vi "Read_Instr.vi"(8 "error in (no error)":errorcluster caption="entrée d'erreur (pas d'erreur)", 11 "Class Instrument Multimeter en entrée":refnum<class "Class Instrument Spectrum_Analyser.lvclass">) -> (0 "error out":errorcluster caption="sortie d'erreur", 3 "Class Instrument Multimeter en sortie":refnum<class "Class Instrument Spectrum_Analyser.lvclass">)   [LabVIEW 2020, in "Library Instrument & Equipement.lvlib" / "Library Instruments.lvlib" / "Class Instrument Spectrum_Analyser.lvclass"]
uses:
  Class Instrument Spectrum_Analyser.lvclass
  Class Instrument Spectrum_Analyser.lvclass/Class Instrument Spectrum_Analyser.ctl
  Instrument (Default)/Class Instrument (Default).lvclass
  Spectrum Analyser/Class Spectrum Analyser (Default)/Class Spectrum Analyser (Default).lvclass
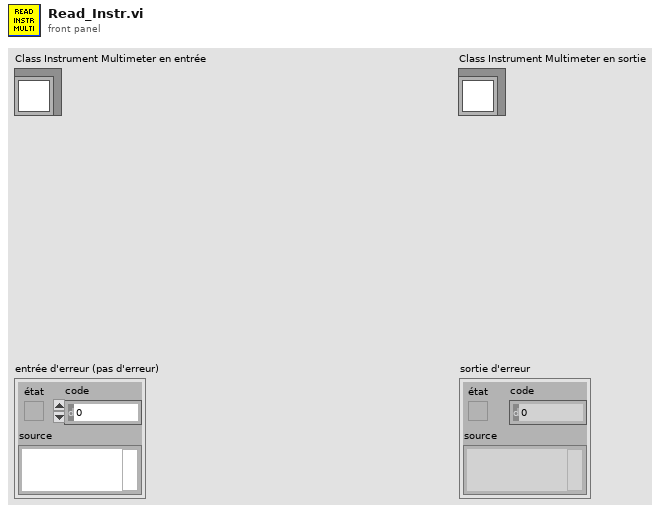
[diagram p1: front panel]
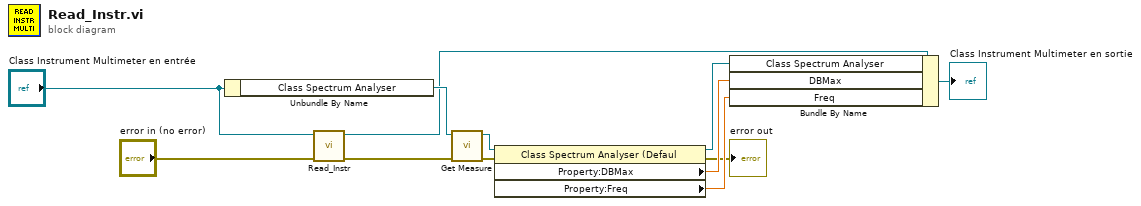
[diagram p0: block diagram]
diagram:
  n1 = Unbundle By Name("Class Instrument Multimeter en entrée") -> ("Class Spectrum Analyser"=w9:refnum<class "Class Spectrum Analyser (Default).lvclass">)
  n2 = call-parent "Read_Instr.vi"("error in (no error)"="error in (no error)", "Class Instrument (Default) en entrée"="Class Instrument Multimeter en entrée") -> ("error out"=w8:errorcluster, "Class Instrument (Default) en sortie"=w1:refnum<class "Class Instrument Spectrum_Analyser.lvclass">)  [unwired: 8 in]
  n3 = call-dynamic "Get Measure.vi"("error in (no error)"=w8, "Class Spectrum Analyser (Default) en entrée"=w9) -> ("error out"=w3:errorcluster, "Class Spectrum Analyser (Default) en sortie"=w7:refnum<class "Class Spectrum Analyser (Default).lvclass">)  [unwired: 8 in]
  n4 = property class="Class Spectrum Analyser (Defaul"(reference=w7, error in=w3) -> (reference out=w6:refnum<class "Class Spectrum Analyser (Default).lvclass">, error out=→"error out":errorcluster, "Property:DBMax"=w5:dbl, "Property:Freq"=w4:dbl)
  n5 = Bundle By Name(cluster=w1, "Class Spectrum Analyser"=w6, "DBMax"=w5, "Freq"=w4) -> (→"Class Instrument Multimeter en sortie":refnum<class "Class Instrument Spectrum_Analyser.lvclass">)
